vi "Draw Filled Star.vi"(6 "Draw Para":T1={"fill?(F)"=TRUE, "color(black)"=0, "pen"={"Width"=1, "Style"=enum."Solid"}}, 8 "错误输入":errorcluster, 10 "Center":T2, 11 "Pic in":picture) -> (0 "错误输出":errorcluster, 3 "Pic out":picture)   [LabVIEW 2011, in "Basic Shape.lvlib"]
uses:
  Point Custom Control.ctl
  Draw Para Custom Control.ctl
  Basic Shape.lvlib
panel:
  in  "Radius":i16=10
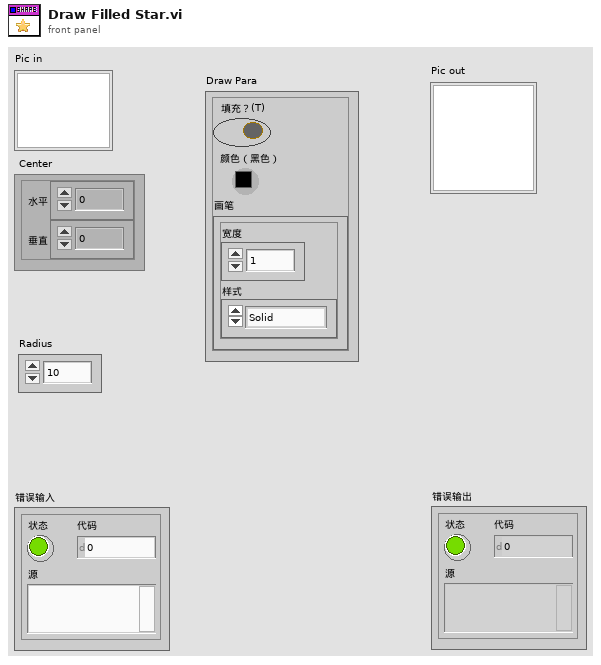
[diagram p1: front panel]
types:
  T1 = typedef "Basic Shape.lvlib/Draw Para Custom Control.ctl" = cluster{"fill?(F)":bool, "color(black)":u32, "pen":cluster{"Width":u16, "Style":enum32{"Solid", "Dash", "Dot", "DashDot", "DashDotDot"}}}
  T2 = typedef "Basic Shape.lvlib/Point Custom Control.ctl" = cluster{"horizontal":i16, "vertical":i16}
  T3 = cluster{"Radius":i16, "Divisions":i16, "Closed":bool}
  T4 = cluster{"Width":u16, "Style":enum32{"Solid", "Dash", "Dot", "DashDot", "DashDotDot"}}
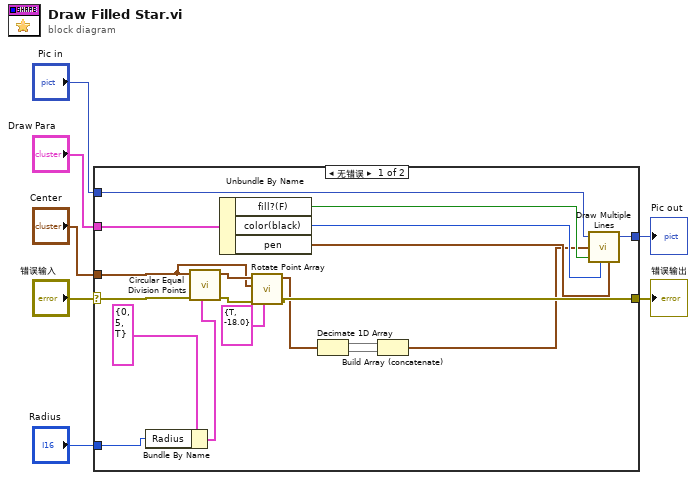
[diagram p0: block diagram]
diagram:
  n1 = case shown="无错误" "错误输入" {
    selector: "错误输入" -> [w26 w28]
    tunnel: [w13 w28] -> w6
    tunnel: "Center" -> [w15 _]
    tunnel: "Pic in" -> [w21 w27]
    tunnel: [w25 w27] -> w3
    tunnel: "Draw Para" -> [w24 _]
    tunnel: "Radius" -> [w18 _]
    frame No Error {
      n2 = Bundle By Name(cluster=T3 {"Radius"=0, "Divisions"=5, "Closed"=TRUE} ("Para"), "Radius"=w18) -> (w17:T3)
      n3 = call "Circular Equal Division Points.vi"("Para"=w17, "错误输入"=w26, "Center"=w15) -> ("错误输出"=w14:errorcluster, "Absolute Point Array"=w16:T2[])  [unwired: 6 in, 1 out]
      n4 = Unbundle By Name(w24) -> ("fill?(F)"=w20:bool, "color(black)"=w22:u32, "pen"=w23:T4)
      n5 = call "Rotate Point Array.vi"("Para"=cluster{"Absolute?":bool, "Angle":dbl} {"Absolute?"=TRUE, "Angle"=-18.0}, "错误输入"=w14, "Center"=w15, "Point Array"=w16) -> ("错误输出"=w13:errorcluster, "Rotated Absolute Point Array"=w8:T2[])  [unwired: 5 in, 1 out]
      n6 = Decimate 1D Array(w8) -> (w11:T2[], w10:T2[])
      n7 = Build Array (concatenate)(w11, w10) -> (w9:T2[])
      n8 = call <vilib>:"Draw Multiple Lines.vi"("picture"=w21, "line endpoints"=w9, "fill?(F)"=w20, "color(black)"=w22, "pen"=w23) -> ("new picture"=w25:picture)  [unwired: 4 in]
    }
    frame Error {
    }
  }
  "Pic out" <- w3
  "错误输出" <- w6
